vi "qam_simulation.vi"() -> ()   [LabVIEW 2020]
uses:
  <vilib>/addons/Modulation/Digital/General/MT Generate Bits (Galois, PN Order).vi
  <vilib>/addons/Modulation/Digital/Support/Common/Validators/mod_Generate Bits Validate.vi
  <vilib>/addons/Modulation/Analog/support/mod_Set Error Source.vi
  <vilib>/addons/Modulation/Digital/Support/Common/Validators/mod_AWGN Validate.vi
  <vilib>/addons/Modulation/Digital/Impairments/subVIs/mod_createSeeds.vi
  <vilib>/addons/Modulation/Digital/Support/Common/Validators/mod_Validate Samples Per Symbol.vi
  <vilib>/addons/Modulation/Analog/support/Validators/mod_Validate Complex Waveform.vi
  <vilib>/addons/Modulation/Analog/support/Validators/mod_WFErrorHandler.vi
  <vilib>/addons/Modulation/Digital/General/MT Generate QAM System Parameters(M).vi
  <vilib>/addons/Modulation/Digital/General/subVIs/mod_Generate Bits PN Sequence.vi
  <vilib>/addons/Modulation/Digital/Support/Common/Validators/mod_Generate Filter Coefficients Validate.vi
  <vilib>/addons/Modulation/Digital/General/subVIs/mod_Generate Filter Coefficients.vi
  <vilib>/Analysis/1siggen.llb/Gaussian White Noise (obs 90).vi
  <vilib>/addons/Modulation/niDMT.lvlib
panel:
  in  "M-QAM (16)":i32=16
  in  "pulse shaping filter (none)":T1(ring)
  in  "Eb/N0 (10 dB)":dbl=10.0 format="%.2f"
  in  "symbol rate (Hz)":dbl=1.0 format="%.2f"
  out "XY Graph":T2(graph)
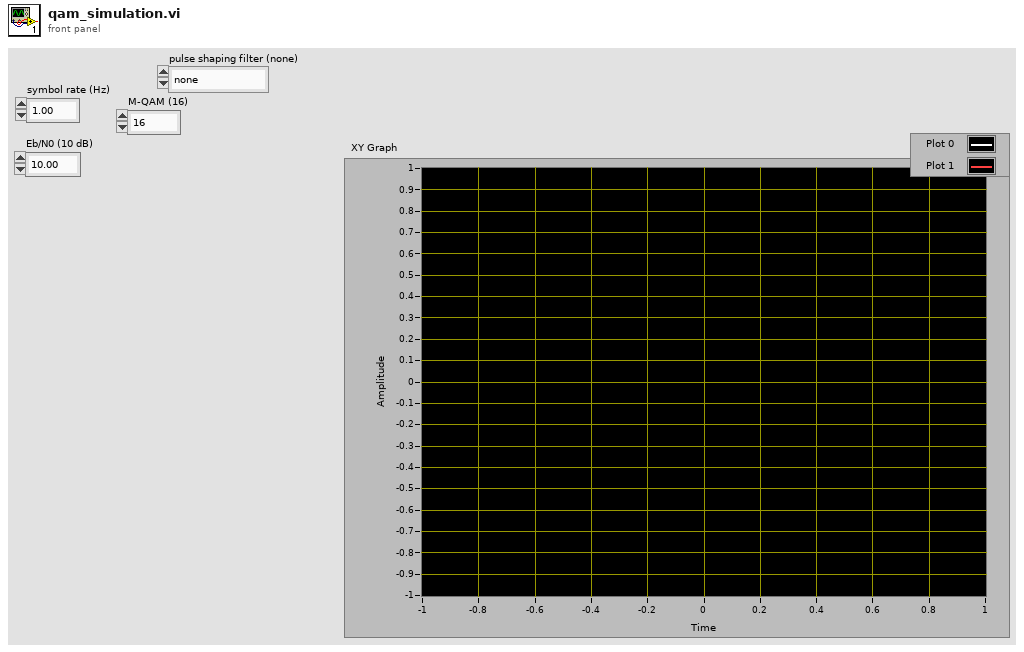
[diagram p1: front panel]
types:
  T1 = enum16{"none", "Raised Cosine", "Root Raised Cos", "Gaussian"}
  T2 = cluster{"constellation":dbl[], "oversampled data":dbl[]}[]
  T3 = enum16{"FSK", "PSK", "QAM", "MSK", "PAM", "ASK", "CPM"}
  T4 = cluster{"samples per symbol (16)":i32, "symbol map":cdb[]}
  T5 = typedef "niAMT.lvlib/Complex Data Waveform.ctl" = cluster{"t0":dbl, "dt":dbl, "Y":cdb[]}
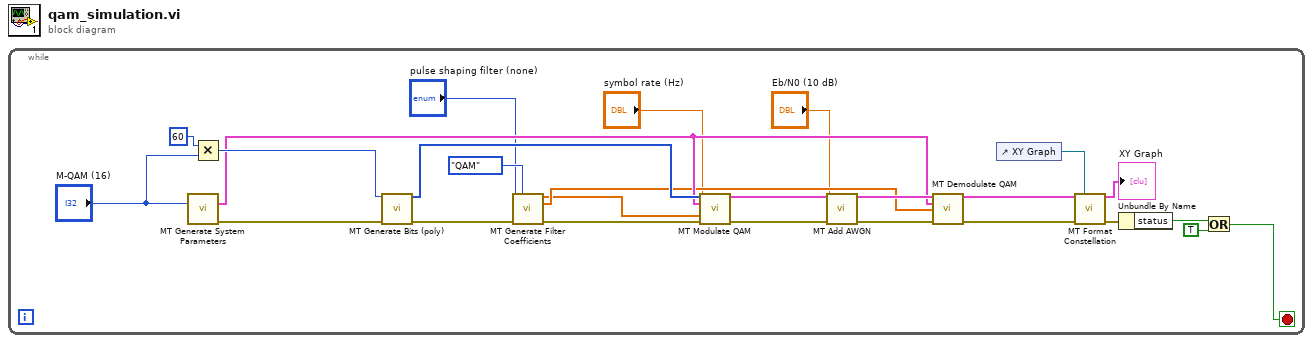
[diagram p0: block diagram]
diagram:
  n1 = while {
    stop <- w3 stop-if-true
    n2 = call-poly <vilib>:"MT Generate System Parameters.vi"("M-QAM (16)"="M-QAM (16)") -> ("QAM system parameters"=w10:T4, "error out"=w16:errorcluster)  [unwired: 12 in, 1 out]
    n3 = Multiply(x=60, y="M-QAM (16)") -> (x*y=w15:i32)
    n4 = call-poly <vilib>:"MT Generate Bits (poly).vi"("total bits (128)"=w15, "error in (no error)"=w16) -> ("output bit stream"=w14:i8[], "error out"=w26:errorcluster)  [unwired: 11 in, 1 out]
    n5 = call <vilib>:"MT Generate Filter Coefficients.vi"("pulse shaping filter (none)"="pulse shaping filter (none)", "modulation type"=T3."QAM", "error in (no error)"=w26) -> ("pulse shaping filter coefficients"=w6:dbl[], "matched filter coefficients"=w9:dbl[], "error out"=w25:errorcluster)  [unwired: 10 in]
    n6 = call <vilib>:"MT Modulate QAM.vi"("input bit stream"=w14, "QAM system parameters"=w10, "symbol rate (Hz)"="symbol rate (Hz)", "pulse shaping filter coefficients"=w6, "error in (no error)"=w25) -> ("output complex waveform"=w13:T5, "error out"=w24:errorcluster)  [unwired: 8 in, 1 out]
    n7 = call <vilib>:"MT Add AWGN.vi"("input complex waveform"=w13, "Eb/N0 (10 dB)"="Eb/N0 (10 dB)", "error in (no error)"=w24) -> ("output complex waveform"=w12:T5, "error out"=w23:errorcluster)  [unwired: 10 in, 1 out]
    n8 = call <vilib>:"MT Demodulate QAM.vi"("input complex waveform"=w12, "QAM system parameters"=w10, "matched filter coefficients"=w9, "error in (no error)"=w23) -> ("recovered complex waveform"=w11:T5, "error out"=w22:errorcluster)  [unwired: 7 in, 3 out]
    n9 = control-ref of="XY Graph"() -> (w20:refnum<vi>)
    n10 = call <vilib>:"MT Format Constellation.vi"("waveform"=w11, "constellation reference"=w20, "error in (no error)"=w22) -> ("constellation graph"=→"XY Graph":T2, "error out"=w19:errorcluster)  [unwired: 11 in]
    n11 = Unbundle By Name(w19) -> ("status"=w18:bool)
    n12 = Or(x=w18, y=TRUE) -> (x .or. y?=w3:bool)
  }
